vi "Example.vi"() -> ()   [LabVIEW 2020]
uses:
  Drivers-IT-M3400/IT-M3400.lvlib
panel:
  in  "Number of Cycles":i32
  in  "Charge filepath":path
  in  "Discharge filepath":path
  in  "Batteryname":string
  in  "Starting Cycle":i32
  out "PS error out":errorcluster
  out "PS Visa Out":refnum<visa-resource-name>
  in  "Wait time":dbl
  in  "Discharge Current Setpoint":dbl format="%#.6g"
  in  "Charge Current Setpoint":dbl format="%#.6g"
  in  "Battery Type":enum16{"\"30Q\"", "\"40T\""}(ring)
  in  "PS error in":errorcluster caption="PS error in (no error)"
  in  "PS VISA in":refnum<visa-resource-name>
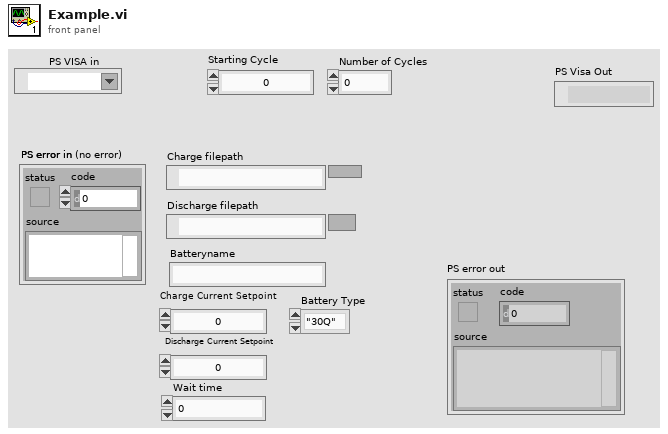
[diagram p1: front panel]
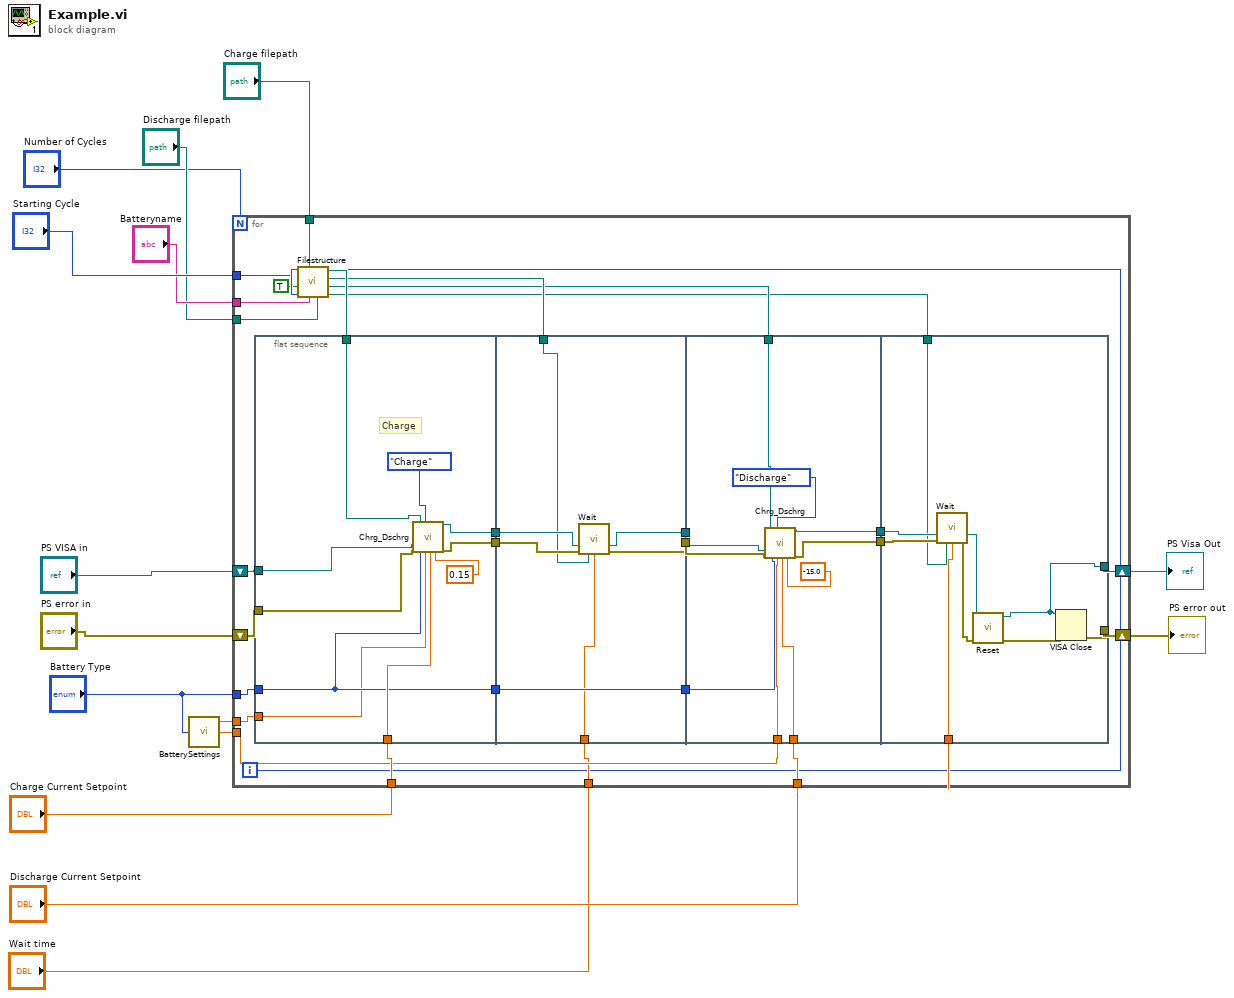
[diagram p0: block diagram]
diagram:
  n1 = call "BatterySettings.vi"("Battery Type"="Battery Type") -> ("Min Voltage (V)"=w10:dbl, "Max Voltage (V)"=w13:dbl)  [unwired: 2 in, 1 out]
  n2 = for {
    N: "Number of Cycles" -> [_]
    tunnel: w13 -> [w33]
    tunnel: "Battery Type" -> [w32]
    tunnel: "Charge Current Setpoint" -> [w31]
    tunnel: w10 -> [w30]
    tunnel: "Discharge Current Setpoint" -> [w29]
    tunnel: "Wait time" -> [w24]
    shift-right: [w22] -> w6
    shift-left: "PS VISA in" -> [w35]
    shift-right: [w23] -> w7
    shift-left: "PS error in" -> [w34]
    tunnel: "Starting Cycle" -> [w20]
    tunnel: "Batteryname" -> [w18]
    tunnel: "Discharge filepath" -> [w17]
    tunnel: "Charge filepath" -> [w16]
    i -> [w21]
    n3 = flat-sequence {
      tunnel: w35 -> [w49]
      tunnel: w34 -> [w48]
      tunnel: w32 -> [w45]
      tunnel: w33 -> [w44]
      tunnel: w31 -> [w46]
      tunnel: [w51] -> w43
      tunnel: [w50] -> w42
      tunnel: [w45] -> w41
      tunnel: w28 -> [w53]
      tunnel: w43 -> [w59]
      tunnel: w42 -> [w58]
      tunnel: [w54] -> w40
      tunnel: [w55] -> w39
      tunnel: w41 -> [w60]
      tunnel: [w60] -> w38
      tunnel: w27 -> [w57]
      tunnel: w24 -> [w56]
      tunnel: w40 -> [w65]
      tunnel: w39 -> [w66]
      tunnel: w38 -> [w67]
      tunnel: w30 -> [w68]
      tunnel: w29 -> [w69]
      tunnel: w26 -> [w61]
      tunnel: [w63] -> w37
      tunnel: [w64] -> w36
      tunnel: w25 -> [w73]
      tunnel: w37 -> [w78]
      tunnel: w36 -> [w77]
      tunnel: w24 -> [w74]
      tunnel: [w79] -> w23
      tunnel: [w72] -> w22
      frame #0 {
        # "Charge"
        n4 = call "Chrg_Dschrg.vi"("PS VISA in"=w49, "PS error in"=w48, "CyclePath"=w53, "Battery Type"=w45, "Charge/discharge"=enum8{"Charge", "Discharge"}."Charge", "Charge/Discharge Voltage Setpoint"=w44, "Current Setpoint"=w46, "Current Cutoff"=0.15) -> ("PS VISA out"=w51:refnum<visa-resource-name>, "PS error out"=w50:errorcluster)  [unwired: 10 in]
      }
      frame #1 {
        n5 = call "Wait.vi"("PS VISA in"=w59, "PS error in"=w58, "Wait Filepath"=w57, "Wait time"=w56) -> ("PS Visa Out"=w54:refnum<visa-resource-name>, "PS error out"=w55:errorcluster)  [unwired: 10 in]
      }
      frame #2 {
        n6 = call "Chrg_Dschrg.vi"("PS VISA in"=w65, "PS error in"=w66, "CyclePath"=w61, "Battery Type"=w67, "Charge/discharge"=enum8{"Charge", "Discharge"}."Discharge", "Charge/Discharge Voltage Setpoint"=w68, "Current Setpoint"=w69, "Current Cutoff"=-15.0) -> ("PS VISA out"=w63:refnum<visa-resource-name>, "PS error out"=w64:errorcluster)  [unwired: 10 in]
      }
      frame #3 {
        n7 = call "Wait.vi"("PS VISA in"=w78, "PS error in"=w77, "Wait Filepath"=w73, "Wait time"=w74) -> ("PS Visa Out"=w76:refnum<visa-resource-name>, "PS error out"=w75:errorcluster)  [unwired: 10 in]
        n8 = call "Reset.vi"("error in"=w75, "VISA resource name"=w76) -> ("error out"=w71:errorcluster, "VISA resource name out"=w72:refnum<visa-resource-name>)  [unwired: 8 in]
        n9 = VISA Close(VISA resource name=w72, error in (no error)=w71) -> (error out=w79:errorcluster)
      }
    }
    n10 = call "Filestructure.vi"("Discharge filepath"=w17, "Batteryname"=w18, "Charge filepath"=w16, "For loop i"=w21, "In for loop"=TRUE, "Starting Cycle"=w20) -> ("DischargeWaitPath"=w25:path, "DischargeCyclePath"=w26:path, "ChargeWaitPath"=w27:path, "ChargeCyclePath"=w28:path)  [unwired: 1 in, 1 out]
  }
  "PS error out" <- w7
  "PS Visa Out" <- w6
